vi "TH_Main.vi"() -> ()   [LabVIEW 2014]
uses:
  TH_Ini_Parameters.vi
  TH_Globals.vi
  TH_StartParameters.vi
panel:
  in  "Main Tab Control":T1(tab)
  in  "Visa logbok":bool
  out "Loggbok":string
  out "FuktCluster":T2={"Fukt 1 (%)"=nan, "Fukt 2 (%)"=nan, "Fukt 3 (%)"=nan} {"Fukt 3 (%)" format="%.1f"; "Fukt 2 (%)" format="%.1f"; "Fukt 1 (%)" format="%.1f"}
  out "TempCluster":T3={"Temp 1 (°C)"=nan, "Temp 2 (°C)"=nan, "Temp 3 (°C)"=nan} {"Temp 3 (°C)" format="%.1f"; "Temp 2 (°C)" format="%.1f"; "Temp 1 (°C)" format="%.1f"}
  out "Tid/Datum":string
  out "Read":bool
  out "TimeDateCluster":T4
  out "Tid/Datum Temp":string
  out "Medeltemp 3":dbl=nan format="%.1f"
  out "Medeltemp 2":dbl=nan format="%.1f"
  out "Medeltemp 1":dbl=nan format="%.1f"
  out "TempXY":T5(graph)
  out "Tid/Datum Fukt":string
  out "Medelfukt 3":dbl=nan format="%.1f"
  out "Medelfukt 2":dbl=nan format="%.1f"
  out "Medelfukt 1":dbl=nan format="%.1f"
  out "FuktXY":T5(graph)
  in  "Medelvärdes-\nbildning":u16(ring) items=["Ingen", "Dynamisk", "6 timmar", "24 timmar"]
  in  "Läs in data":bool
  in  "Slut Dag":u16(ring) items=["1", "2", "3", "4", "5", "6", "7", "8", "9", "10", "11", "12", "13", "14", "15", "16", "17", "18", "19", "20", "21", "22", "23", "24", "25", "26", "27", "28", "29", "30", "31"]
  in  "Slut Månad":u16(ring) items=["Januari", "Februari", "Mars", "April", "Maj", "Juni", "Juli", "Augusti", "September", "Oktober", "November", "December"]
  in  "Slut År":u16(ring)=4 items=["2001", "2002", "2003", "2004", "2005", "2006", "2007", "2008", "2009", "2010", "2011", "2012", "2013", "2014", "2015"]
  in  "Start Dag":u16(ring) items=["1", "2", "3", "4", "5", "6", "7", "8", "9", "10", "11", "12", "13", "14", "15", "16", "17", "18", "19", "20", "21", "22", "23", "24", "25", "26", "27", "28", "29", "30", "31"]
  in  "Start Månad":u16(ring) items=["Januari", "Februari", "Mars", "April", "Maj", "Juni", "Juli", "Augusti", "September", "Oktober", "November", "December"]
  in  "Start År":u16(ring)=4 items=["2001", "2002", "2003", "2004", "2005", "2006", "2007", "2008", "2009", "2010", "2011", "2012", "2013", "2014", "2015"]
  out "XY Graph":T6(graph)
  in  "Starta backup":bool
  in  "Backup år":u16(ring)=4 items=["2001", "2002", "2003", "2004", "2005", "2006", "2007", "2008", "2009", "2010"]
  in  "Bladmögel":T7={"Tid (timmar)"=4.0, "Temp (°C)"=3.0, "Fukt (%)"=93.0} {"Fukt (%)" min=0.0 max=100.0 format="%.1f"; "Temp (°C)" min=-25.0 max=85.0 step=0.1 format="%.1f"; "Tid (timmar)" min=0.01 format="%.2f"}
  in  "MainExit":bool
  in  "Skriv ut skärmbild":bool
  # "Från:"
  # "Till:"
  # "Backup av mätdata\ntill diskett A:\\"
  # "Bladmögelvarning\nför givare 1"
  # "TH-Logger är ett svenskutvecklat program som visar och lagrar temperatur och fukt information om förhållandena i vilka lagerutrymmen som helst.\n\nProgrammet är utvecklat av Roine Stenberg och Niklas Jonsson och har varit i drift och utvecklats sedan hösten 2001, bland annat i Niklas Jonssons eget lager på Follinge Krongård.\n\nMer information om programmet och hur det kan användas får du genom att ringa Niklas Jonsson på telefon 0142-41749 eller 0708-441749. Tekniska frågor besvaras av Roine Stenberg på telefon 013-105646 eller 0733-253321.\n\nPå internet finns också en del information om programmet på adressen http://www.follinge.se"
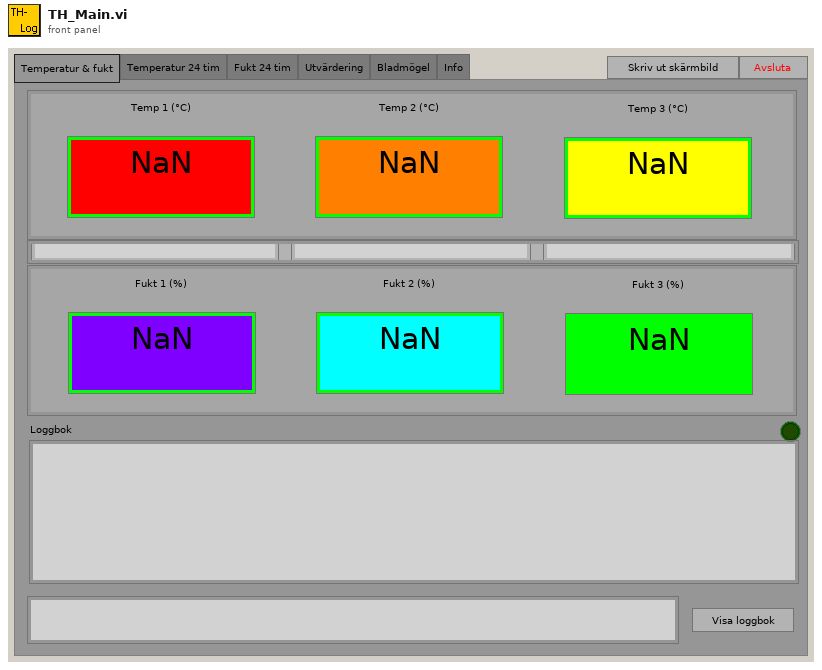
[diagram p1: front panel]
types:
  T1 = enum32{"Temperatur & fukt", "Temperatur 24 tim", "Fukt 24 tim", "Utvärdering", "Bladmögel", "Info"}
  T2 = cluster{"Fukt 1 (%)":dbl, "Fukt 2 (%)":dbl, "Fukt 3 (%)":dbl}
  T3 = cluster{"Temp 1 (°C)":dbl, "Temp 2 (°C)":dbl, "Temp 3 (°C)":dbl}
  T4 = cluster{"TimeDate 1":string, "TimeDate 2":string, "TimeDate 3":string}
  T5 = cluster{"XY chart data":cluster{"x":dbl, "y":dbl}[]}[]
  T6 = cluster{cluster{"Numeric":dbl, "Numeric":dbl}[]}[]
  T7 = cluster{"Tid (timmar)":dbl, "Temp (°C)":dbl, "Fukt (%)":dbl}
  T8 = cluster{"Temperatures[0]":dbl, "Temperatures[1]":dbl, "Temperatures[2]":dbl}
  T9 = cluster{"Humidities[0]":dbl, "Humidities[1]":dbl, "Humidities[2]":dbl}
  T10 = typedef "NH485 Object Reference.ctl" = refnum<k1>
  T11 = cluster{"[0]":string, "[1]":string, "[2]":string}
  T12 = cluster{"Start År":u16, "Start Månad":u16, "Start Dag":u16, "Slut År":u16, "Slut Månad":u16, "Slut Dag":u16}
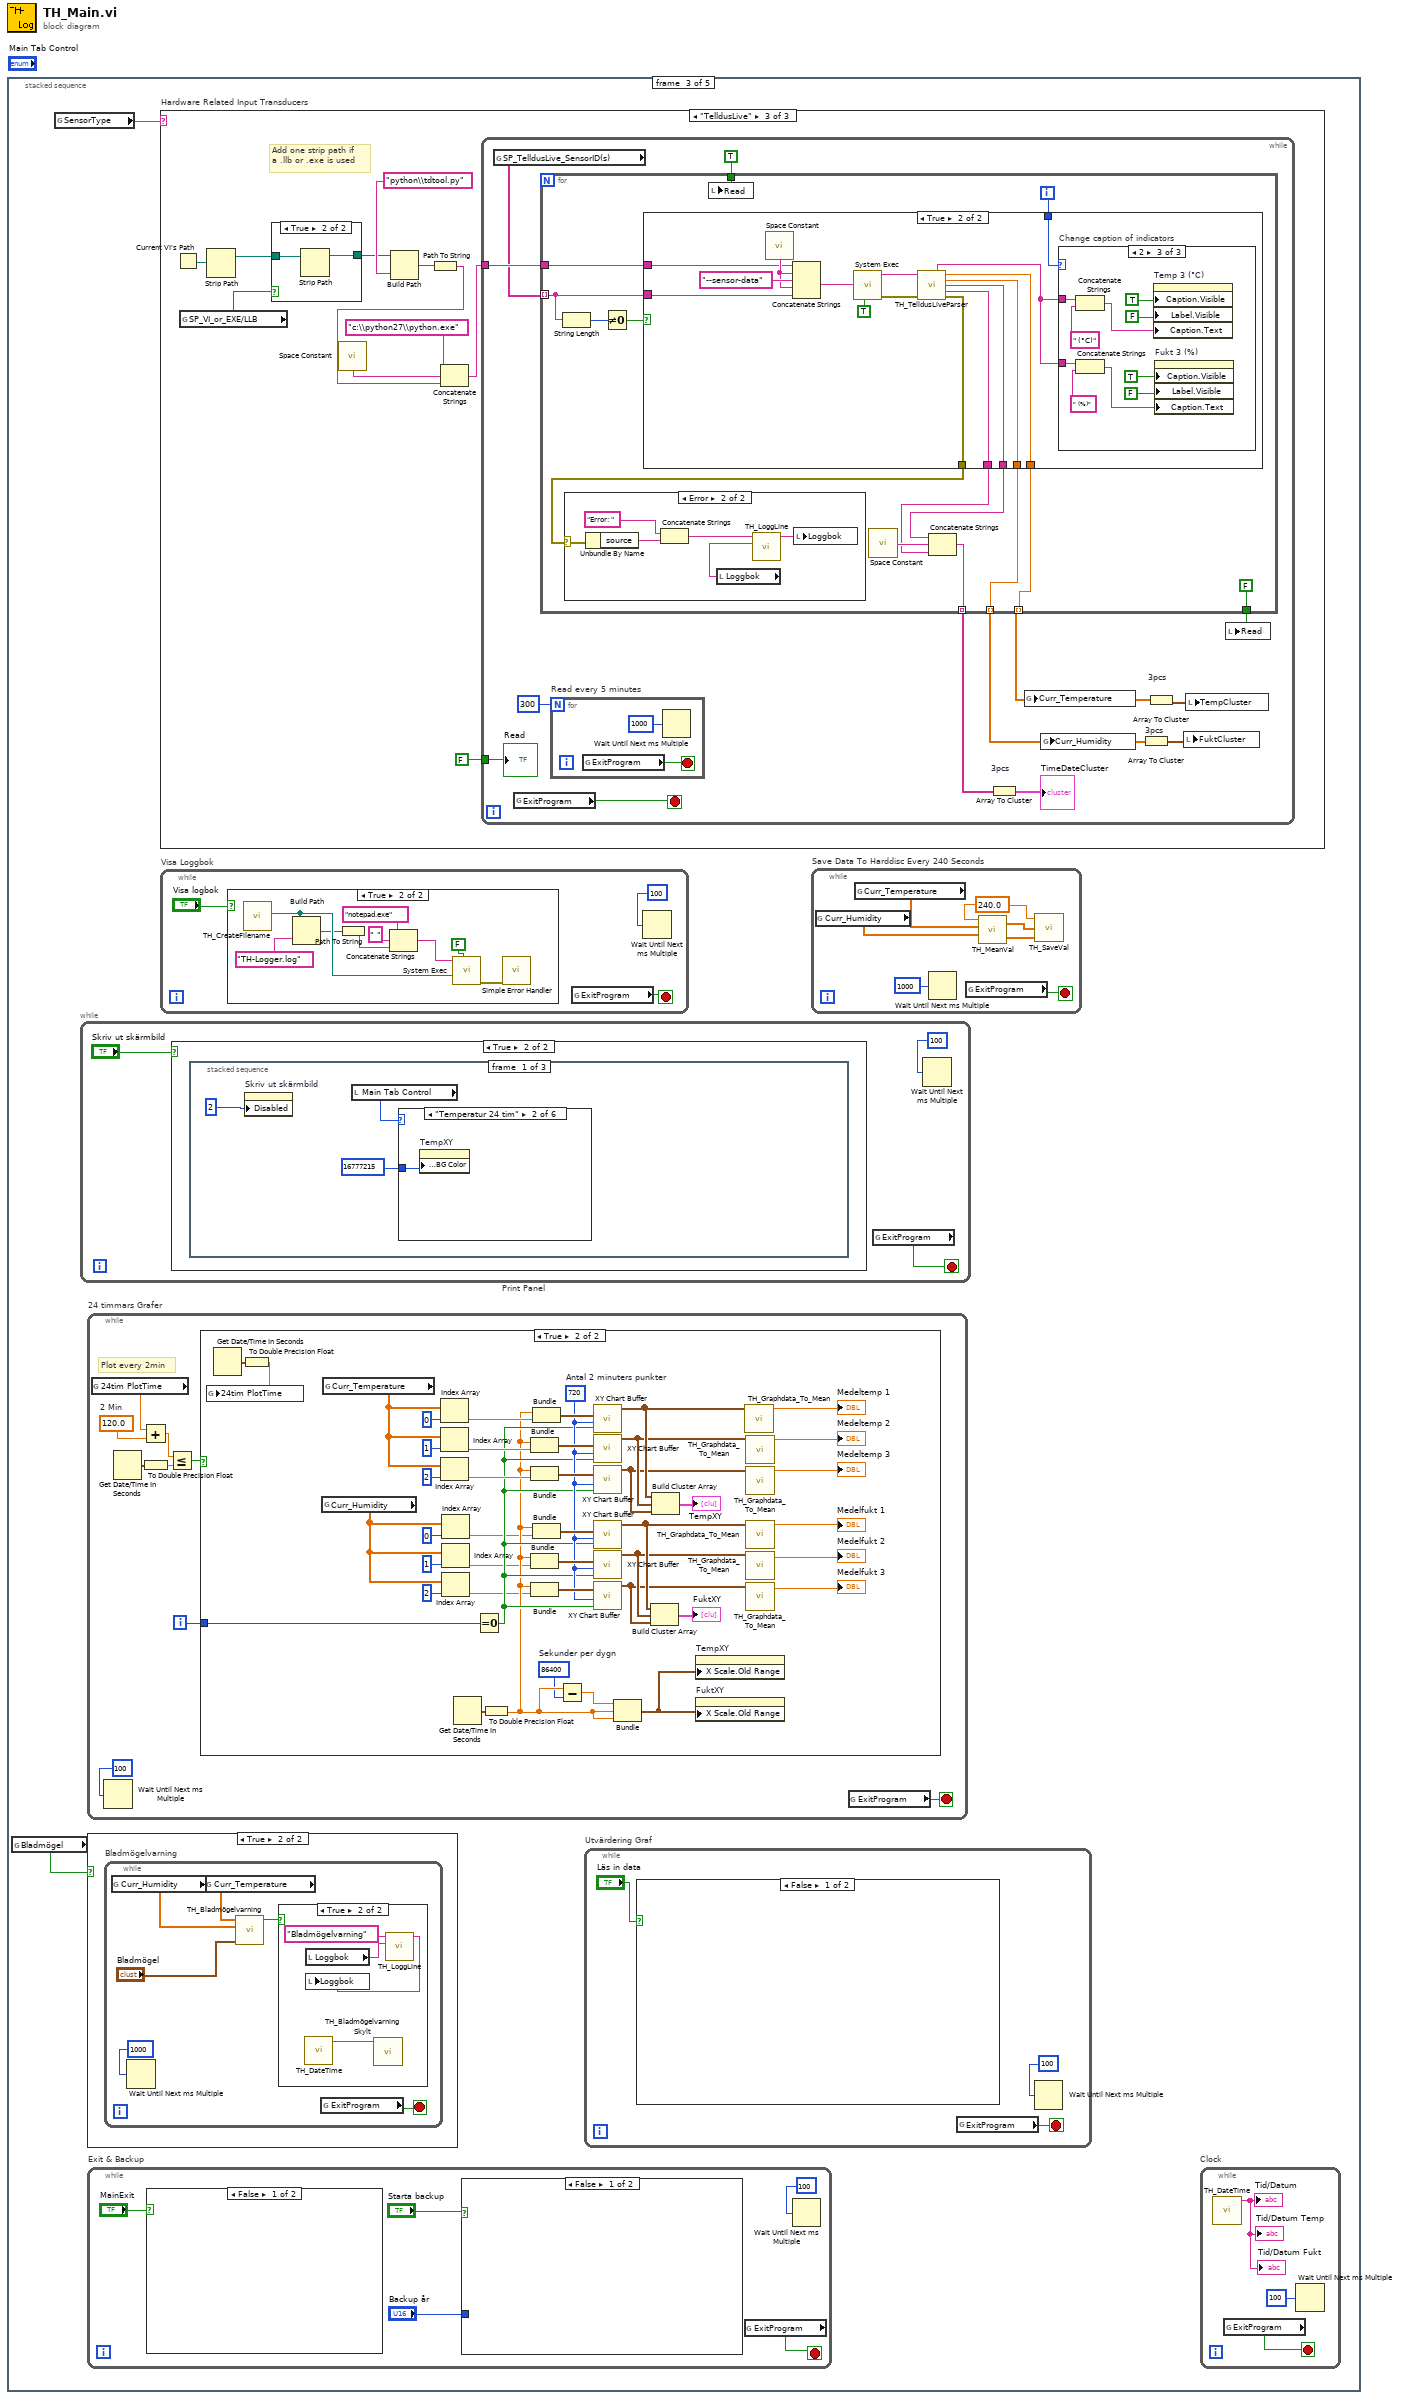
[diagram p0: block diagram]
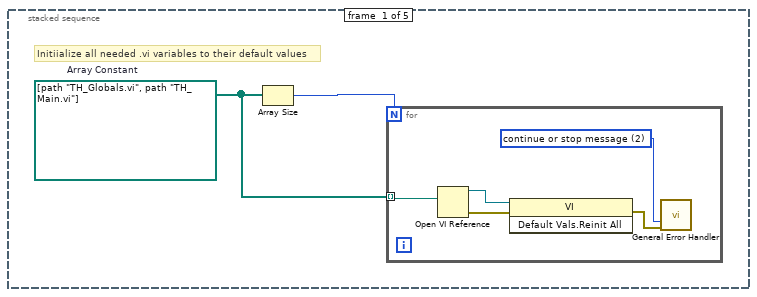
[diagram p2: hidden frame]
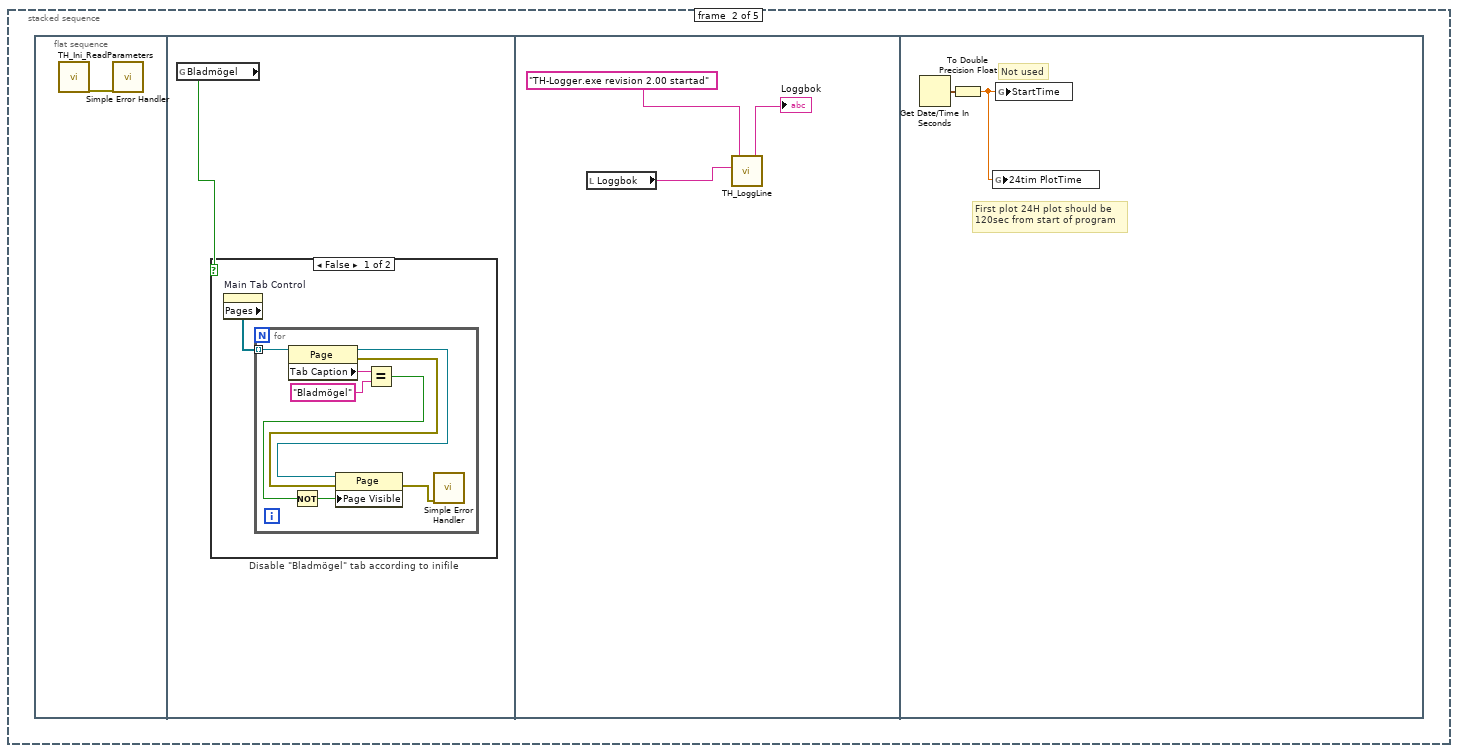
[diagram p3: hidden frame]
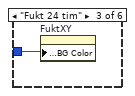
[diagram p10: hidden frame]
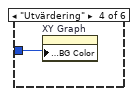
[diagram p11: hidden frame]
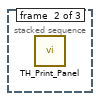
[diagram p14: hidden frame]
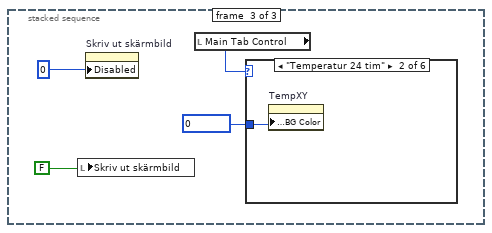
[diagram p15: hidden frame]
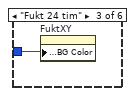
[diagram p17: hidden frame]
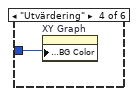
[diagram p18: hidden frame]
diagram:
  n1 = stacked-sequence {
    frame #0 {
      w1 = path[] [path "TH_Globals.vi", path "TH_Main.vi"]  # Array Constant
      # "Initiialize all needed .vi variables to their default values"
      n2 = Array Size(array=w1) -> (size(s)=w2:i32)
      n3 = for {
        N: w2 -> [_]
        tunnel: w1 -> [w7] mode=indexing
        w3 = u16 2 items=["no dialog", "OK message", "continue or stop message"] ("type of dialog (OK msg:1)")
        n4 = Open VI Reference(vi path=w7) -> (vi reference=w5:refnum<vi>, error out=w6:errorcluster)  [unwired: 5 in]
        n5 = invoke class="VI" method="Default Vals.Reinit All"(reference=w5, error in=w6) -> (error out=w4:errorcluster)  [unwired: 1 in, 2 out]
        n6 = call <vilib>:"General Error Handler.vi"("type of dialog (OK msg:1)"=w3, "error in (no error)"=w4) -> ()  [unwired: 9 in, 5 out]
      }
    }
    frame #1 {
      n7 = flat-sequence {
        frame #0 {
          n8 = call "TH_Ini_ReadParameters.vi"() -> ("error out"=w8:errorcluster)  [unwired: 19 in]
          n9 = call <vilib>:"Simple Error Handler.vi"("error in (no error)"=w8) -> ()  [unwired: 4 in, 5 out]
        }
        frame #1 {
          n10 = global read "TH_Ini_Parameters.vi" "Bladmögel"() -> (w9:bool)
          n11 = case "Disable \"Bladmögel\" tab according to inifile" shown="False" w9 {
            frame False {
              n12 = property on="Main Tab Control" class="TabCtl (strict)"() -> ("Pages"=w10:refnum<vi>[])  [unwired: 2 in, 2 out]
              n13 = for {
                tunnel: w10 -> [w18] mode=indexing
                n14 = property class="Page"(reference=w18) -> (reference out=w14:refnum<vi>, error out=w15:errorcluster, "Tab Caption"=w17:string)  [unwired: 1 in]
                n15 = Equal?(x=w17, y="Bladmögel") -> (x = y?=w12:bool)
                n16 = Not(x=w12) -> (.not. x?=w11:bool)
                n17 = property class="Page"(reference=w14, error in=w15, "Page Visible"=w11) -> (error out=w13:errorcluster)  [unwired: 1 out]
                n18 = call <vilib>:"Simple Error Handler.vi"("error in (no error)"=w13) -> ()  [unwired: 4 in, 5 out]
              }
            }
            frame True {
            }
          }
        }
        frame #2 {
          n19 = local read "Loggbok"() -> (w21:string)
          n20 = call "TH_LoggLine.vi"("Händelse Logg In"=w21, "Logg String In"="TH-Logger.exe revision 2.00 startad") -> ("Händelse Logg Out"=→"Loggbok":string)  [unwired: 5 in]
        }
        frame #3 {
          # "Not used"
          # "First plot 24H plot should be\n120sec from start of program"
          n21 = Get Date/Time In Seconds() -> (seconds since 1Jan1904=w23:timestamp)
          n22 = To Double Precision Float(number=w23) -> (double precision float=w22:dbl)
          n23 = global write "TH_Globals.vi" "24tim PlotTime"(w22) -> ()
          n24 = global write "TH_Globals.vi" "StartTime"(w22) -> ()
        }
      }
    }
    frame #2 {
      n25 = global read "TH_Ini_Parameters.vi" "Bladmögel"() -> (w24:bool)
      n26 = global read "TH_Ini_Parameters.vi" "SensorType"() -> (w25:string)
      n27 = while "Print Panel" {
        stop <- w49 stop-if-true
        n28 = case shown="True" "Skriv ut skärmbild" {
          frame False {
          }
          frame True {
            n29 = stacked-sequence {
              frame #0 {
                n30 = property on="Skriv ut skärmbild" class="Bool (strict)"("Disabled"=2) -> ()  [unwired: 2 in, 2 out]
                n31 = local read "Main Tab Control"() -> (w52:T1)
                n32 = case shown="\"Temperatur 24 tim\"" w52 {
                  tunnel: u32 16777215 ("Plot Area:Colors:BG Color") -> [_ w54 w55 w56 _ _]
                  frame "Temperatur & fukt", Default {
                  }
                  frame "Temperatur 24 tim" {
                    n33 = property on="TempXY" class="XYGraph (strict)"("Plot Area:Colors:BG Color"=w54) -> ()  [unwired: 2 in, 2 out]
                  }
                  frame "Fukt 24 tim" {
                    n34 = property on="FuktXY" class="XYGraph (strict)"("Plot Area:Colors:BG Color"=w55) -> ()  [unwired: 2 in, 2 out]
                  }
                  frame "Utvärdering" {
                    n35 = property on="XY Graph" class="XYGraph (strict)"("Plot Area:Colors:BG Color"=w56) -> ()  [unwired: 2 in, 2 out]
                  }
                  frame "Bladmögel" {
                  }
                  frame "Info" {
                  }
                }
              }
              frame #1 {
                n36 = call "TH_Print_Panel.vi"() -> ()  [unwired: 20 in]
              }
              frame #2 {
                n37 = local write "Skriv ut skärmbild"(FALSE) -> ()
                n38 = property on="Skriv ut skärmbild" class="Bool (strict)"("Disabled"=0) -> ()  [unwired: 2 in, 2 out]
                n39 = local read "Main Tab Control"() -> (w58:T1)
                n40 = case shown="\"Temperatur 24 tim\"" w58 {
                  tunnel: u32 0 ("Plot Area:Colors:BG Color") -> [_ w61 w62 w63 _ _]
                  frame "Temperatur & fukt", Default {
                  }
                  frame "Temperatur 24 tim" {
                    n41 = property on="TempXY" class="XYGraph (strict)"("Plot Area:Colors:BG Color"=w61) -> ()  [unwired: 2 in, 2 out]
                  }
                  frame "Fukt 24 tim" {
                    n42 = property on="FuktXY" class="XYGraph (strict)"("Plot Area:Colors:BG Color"=w62) -> ()  [unwired: 2 in, 2 out]
                  }
                  frame "Utvärdering" {
                    n43 = property on="XY Graph" class="XYGraph (strict)"("Plot Area:Colors:BG Color"=w63) -> ()  [unwired: 2 in, 2 out]
                  }
                  frame "Bladmögel" {
                  }
                  frame "Info" {
                  }
                }
              }
            }
          }
        }
        n44 = global read "TH_Globals.vi" "ExitProgram"() -> (w49:bool)
        n45 = Wait Until Next ms Multiple(millisecond multiple=u32 100) -> ()  [unwired: 1 out]
      }
      n46 = while "24 timmars Grafer" {
        i -> [w72]
        stop <- w65 stop-if-true
        w68 = 120.0  # 2 Min
        # "Plot every 2min"
        n47 = global read "TH_Globals.vi" "24tim PlotTime"() -> (w67:dbl)
        n48 = Wait Until Next ms Multiple(millisecond multiple=u32 100) -> ()  [unwired: 1 out]
        n49 = Get Date/Time In Seconds() -> (seconds since 1Jan1904=w64:timestamp)
        n50 = Add(x=w67, y=w68) -> (x+y=w69:dbl)
        n51 = To Double Precision Float(number=w64) -> (double precision float=w70:dbl)
        n52 = Less Or Equal?(x=w69, y=w70) -> (x <= y?=w66:bool)
        n53 = case shown="True" w66 {
          tunnel: w72 -> [_ w116]
          frame False {
          }
          frame True {
            w95 = 720  # Antal 2 minuters punkter
            w88 = 86400  # Sekunder per dygn
            n54 = Get Date/Time In Seconds() -> (seconds since 1Jan1904=w73:timestamp)
            n55 = To Double Precision Float(number=w73) -> (double precision float=w115:dbl)
            n56 = global write "TH_Globals.vi" "24tim PlotTime"(w115) -> ()
            n57 = global read "TH_Globals.vi" "Curr_Humidity"() -> (w99:dbl[])
            n58 = global read "TH_Globals.vi" "Curr_Temperature"() -> (w109:dbl[])
            n59 = Index Array(array=w109, index=0) -> (element=w111:dbl)
            n60 = Index Array(array=w109, index=1) -> (element=w110:dbl)
            n61 = Index Array(array=w109, index=2) -> (element=w105:dbl)
            n62 = Index Array(array=w99, index=0) -> (element=w92:dbl)
            n63 = Index Array(array=w99, index=1) -> (element=w91:dbl)
            n64 = Index Array(array=w99, index=2) -> (element=w90:dbl)
            n65 = Get Date/Time In Seconds() -> (seconds since 1Jan1904=w74:timestamp)
            n66 = Equal To 0?(x=w116) -> (x = 0?=w94:bool)
            n67 = To Double Precision Float(number=w74) -> (double precision float=w93:dbl)
            n68 = Bundle(w93, "Numeric"=w110) -> (w112:cluster{dbl, "Numeric":dbl})  [unwired: 1 in]
            n69 = Bundle(w93, "Numeric"=w105) -> (w103:cluster{dbl, "Numeric":dbl})  [unwired: 1 in]
            n70 = Bundle(w93, "Numeric"=w91) -> (w97:cluster{dbl, "Numeric":dbl})  [unwired: 1 in]
            n71 = Bundle(w93, "Numeric"=w90) -> (w98:cluster{dbl, "Numeric":dbl})  [unwired: 1 in]
            n72 = Bundle(w93, "Numeric"=w111) -> (w114:cluster{dbl, "Numeric":dbl})  [unwired: 1 in]
            n73 = Bundle(w93, "Numeric"=w92) -> (w96:cluster{dbl, "Numeric":dbl})  [unwired: 1 in]
            n74 = Subtract(x=w93, y=w88) -> (x-y=w113:dbl)
            n75 = call "XY Chart Buffer.vi"("clear first (no:F)"=w94, "chart length (points)"=w95, "new point"=w114) -> ("XY chart data"=w86:cluster{"x":dbl, "y":dbl}[])  [unwired: 8 in]
            n76 = call "XY Chart Buffer.vi"("clear first (no:F)"=w94, "chart length (points)"=w95, "new point"=w112) -> ("XY chart data"=w85:cluster{"x":dbl, "y":dbl}[])  [unwired: 8 in]
            n77 = call "XY Chart Buffer.vi"("clear first (no:F)"=w94, "chart length (points)"=w95, "new point"=w103) -> ("XY chart data"=w84:cluster{"x":dbl, "y":dbl}[])  [unwired: 8 in]
            n78 = call "XY Chart Buffer.vi"("clear first (no:F)"=w94, "chart length (points)"=w95, "new point"=w96) -> ("XY chart data"=w83:cluster{"x":dbl, "y":dbl}[])  [unwired: 8 in]
            n79 = call "XY Chart Buffer.vi"("clear first (no:F)"=w94, "chart length (points)"=w95, "new point"=w97) -> ("XY chart data"=w82:cluster{"x":dbl, "y":dbl}[])  [unwired: 8 in]
            n80 = call "XY Chart Buffer.vi"("clear first (no:F)"=w94, "chart length (points)"=w95, "new point"=w98) -> ("XY chart data"=w81:cluster{"x":dbl, "y":dbl}[])  [unwired: 8 in]
            n81 = Bundle(w113, w93, w93) -> (w87:cluster{dbl, dbl, dbl})  [unwired: 1 in]
            n82 = Build Cluster Array(w83, w82, w81) -> (→"FuktXY":T5)
            n83 = Build Cluster Array(w86, w85, w84) -> (→"TempXY":T5)
            n84 = property on="TempXY" class="XYGraph (strict)"("X Scale.Old Range"=w87) -> ()  [unwired: 2 in, 2 out]
            n85 = property on="FuktXY" class="XYGraph (strict)"("X Scale.Old Range"=w87) -> ()  [unwired: 2 in, 2 out]
            n86 = call "TH_Graphdata_To_Mean.vi"("XY chart data"=w86) -> ("MeanValue"=→"Medeltemp 1":dbl)  [unwired: 5 in, 1 out]
            n87 = call "TH_Graphdata_To_Mean.vi"("XY chart data"=w85) -> ("MeanValue"=→"Medeltemp 2":dbl)  [unwired: 5 in, 1 out]
            n88 = call "TH_Graphdata_To_Mean.vi"("XY chart data"=w84) -> ("MeanValue"=→"Medeltemp 3":dbl)  [unwired: 5 in, 1 out]
            n89 = call "TH_Graphdata_To_Mean.vi"("XY chart data"=w83) -> ("MeanValue"=→"Medelfukt 1":dbl)  [unwired: 5 in, 1 out]
            n90 = call "TH_Graphdata_To_Mean.vi"("XY chart data"=w82) -> ("MeanValue"=→"Medelfukt 2":dbl)  [unwired: 5 in, 1 out]
            n91 = call "TH_Graphdata_To_Mean.vi"("XY chart data"=w81) -> ("MeanValue"=→"Medelfukt 3":dbl)  [unwired: 5 in, 1 out]
          }
        }
        n92 = global read "TH_Globals.vi" "ExitProgram"() -> (w65:bool)
      }
      n93 = case shown="True" w24 {
        frame False {
        }
        frame True {
          n94 = while "Bladmögelvarning" {
            stop <- w27 stop-if-true
            n95 = global read "TH_Globals.vi" "Curr_Humidity"() -> (w29:dbl[])
            n96 = Wait Until Next ms Multiple(millisecond multiple=u32 1000) -> ()  [unwired: 1 out]
            n97 = global read "TH_Globals.vi" "Curr_Temperature"() -> (w30:dbl[])
            n98 = call "TH_Bladmögelvarning.vi"("Bladmögelvarning"="Bladmögel", "Humidities In"=w29, "Temperatures In"=w30) -> ("Bladmägelvarning (T/F)"=w26:bool)  [unwired: 4 in]
            n99 = case shown="True" w26 {
              frame False {
              }
              frame True {
                n100 = call "TH_DateTime.vi"() -> ("Tid och Datum"=w32:string)  [unwired: 7 in]
                n101 = local read "Loggbok"() -> (w33:string)
                n102 = call "TH_Bladmögelvarning Skylt.vi"("Tid"=w32) -> ()  [unwired: 7 in]
                n103 = call "TH_LoggLine.vi"("Händelse Logg In"=w33, "Logg String In"="Bladmögelvarning") -> ("Händelse Logg Out"=w35:string)  [unwired: 5 in]
                n104 = local write "Loggbok"(w35) -> ()
              }
            }
            n105 = global read "TH_Globals.vi" "ExitProgram"() -> (w27:bool)
          }
        }
      }
      n106 = while "Exit & Backup" {
        stop <- w136 stop-if-true
        n107 = case shown="False" "MainExit" {
          frame False {
          }
          frame True {
            n108 = Two Button Dialog(message="Är du säker på att du vill avsluta detta program?", 1:"Nej" ("F button name (\"Cancel\")"), 2:"Ja" ("T button name (\"OK\")")) -> (T button?=w152:bool)
            n109 = case shown="True" w152 {
              frame False {
              }
              frame True {
                n110 = global write "TH_Globals.vi" "ExitProgram"(TRUE) -> ()
              }
            }
          }
        }
        n111 = case shown="False" "Starta backup" {
          tunnel: "Backup år" -> [_ w139]
          frame False {
          }
          frame True {
            (unwired) "\u001b" ("message")
            n112 = stacked-sequence {
              tunnel: w139 -> [_ w141 _]
              frame #0 {
                n113 = property on="Starta backup" class="Bool (strict)"("Disabled"=2) -> ()  [unwired: 2 in, 2 out]
              }
              frame #1 {
                n114 = Two Button Dialog(message="Placera en formaterad 1.44MB diskett i diskettstation A:\\\nAlla befintliga filer kommer att raderas!", 1:"Avbryt" ("F button name (\"Cancel\")"), 2:"OK" ("T button name (\"OK\")")) -> (T button?=w142:bool)
                n115 = case shown="True" w142 {
                  tunnel: w141 -> [_ w146]
                  frame False {
                  }
                  frame True {
                    n116 = call "TH_DataBackup.vi"("Backup År"=w146) -> ()  [unwired: 5 in, 2 out]
                  }
                }
              }
              frame #2 {
                n117 = local write "Starta backup"(FALSE) -> ()
                n118 = property on="Starta backup" class="Bool (strict)"("Disabled"=0) -> ()  [unwired: 2 in, 2 out]
              }
            }
          }
        }
        n119 = global read "TH_Globals.vi" "ExitProgram"() -> (w136:bool)
        n120 = Wait Until Next ms Multiple(millisecond multiple=u32 100) -> ()  [unwired: 1 out]
      }
      n121 = case "Hardware Related Input Transducers" shown="\"TelldusLive\"" w25 {
        frame "HygroWin", Default {
          n122 = global read "TH_StartParameters.vi" "SP_HygroWin_COMport(s)"() -> (w165:refnum<visa-resource-name>[])
          n123 = call "TH_RS232_Init.vi"("COMports"=w165) -> ("error out array"=w164:errorcluster[], "COMhandles"=w168:refnum<visa-resource-name>[])  [unwired: 5 in]
          n124 = while "Read Port Loop (This should be the fastest routine in the program)" {
            tunnel: [w170] -> w166
            tunnel: w164 -> [w174]
            tunnel: [w177] -> w167
            tunnel: w168 -> [w178]
            stop <- w169 stop-if-true
            n125 = call "TH_RS232_Read.vi"("COMhandles In"=w178, "error in array"=w174) -> ("NewValues Out"=w173:bool[], "COMhandles Out"=w177:refnum<visa-resource-name>[], "Temperatures"=w171:dbl[], "Humidities"=w172:dbl[], "error out array"=w170:errorcluster[])  [unwired: 2 in]
            n126 = global write "TH_Globals.vi" "Curr_Temperature"(w171) -> ()
            n127 = Array To Cluster "3pcs"(array=w171) -> (cluster=→"TempCluster":T8)
            n128 = global write "TH_Globals.vi" "Curr_Humidity"(w172) -> ()
            n129 = global write "TH_Globals.vi" "NewValues"(w173) -> ()
            n130 = Array To Cluster "3pcs"(array=w172) -> (cluster=→"FuktCluster":T9)
            n131 = global read "TH_Globals.vi" "ExitProgram"() -> (w169:bool)
            n132 = Wait Until Next ms Multiple(millisecond multiple=u32 100) -> ()  [unwired: 1 out]
          }
          n133 = for "Create/Open Error Dialog" {
            tunnel: w164 -> [w181] mode=indexing
            i -> [w180]
            n134 = case shown="Error" w181 {
              tunnel: w180 -> [_ w186]
              frame No Error {
              }
              frame Error {
                n135 = Number To Decimal String(number=w186) -> (decimal integer string=w185:string)  [unwired: 1 in]
                n136 = local read "Loggbok"() -> (w184:string)
                n137 = Concatenate Strings("Error, Open VISA Port. Array Position ", w185) -> (w182:string)
                n138 = call "TH_LoggLine.vi"("Händelse Logg In"=w184, "Logg String In"=w182) -> ("Händelse Logg Out"=w183:string)  [unwired: 5 in]
                n139 = local write "Loggbok"(w183) -> ()
              }
            }
          }
          n140 = call "TH_RS232_Exit.vi"("Array"=w166, "COMports"=w167) -> ()  [unwired: 6 in]
        }
        frame "NH485" {
          n141 = global read "TH_StartParameters.vi" "SP_NH485_COMport"() -> (w189:refnum<visa-resource-name>[])
          n142 = global read "TH_StartParameters.vi" "SP_NH485_Adress(es)"() -> (w188:u32[])
          n143 = for "Create/Open" {
            tunnel: w189 -> [w234] mode=indexing
            tunnel: [w231] -> w190 mode=indexing
            tunnel: [w230] -> w191 mode=indexing
            tunnel: w188 -> [w229] mode=indexing
            n144 = call "NH485 Create.vi"("Address"=w229, "VISA Resource Name"=w234) -> ("error out"=w232:errorcluster, "reference"=w233:T10)  [unwired: 4 in]
            n145 = call "NH485 Open.vi"("error in (no error)"=w232, "reference"=w233) -> ("error out"=w230:errorcluster, "duplicate reference"=w231:T10)  [unwired: 8 in]
          }
          n146 = for "Create/Open Error Dialog" {
            tunnel: w191 -> [w218] mode=indexing
            i -> [w217]
            n147 = case shown="Error" w218 {
              tunnel: w217 -> [_ w223]
              frame No Error {
              }
              frame Error {
                n148 = Number To Decimal String(number=w223) -> (decimal integer string=w222:string)  [unwired: 1 in]
                n149 = local read "Loggbok"() -> (w221:string)
                n150 = Concatenate Strings("Error, Open VISA Port. Array Position ", w222) -> (w219:string)
                n151 = call "TH_LoggLine.vi"("Händelse Logg In"=w221, "Logg String In"=w219) -> ("Händelse Logg Out"=w220:string)  [unwired: 5 in]
                n152 = local write "Loggbok"(w220) -> ()
              }
            }
          }
          n153 = while "Read Transducer Data" {
            tunnel: [w195] -> w192
            tunnel: [w196] -> w193
            tunnel: w191 -> [w198]
            tunnel: w190 -> [w199]
            stop <- w194 stop-if-true
            n154 = for {
              tunnel: [w204] -> w195 mode=indexing
              tunnel: [w203] -> w196 mode=indexing
              tunnel: w199 -> [w202] mode=indexing
              tunnel: w198 -> [w201] mode=indexing
              n155 = call "NH485 Measure.vi"("error in (no error)"=w201, "reference"=w202) -> ("error out"=w204:errorcluster, "duplicate reference"=w203:T10)  [unwired: 8 in]
              n156 = Wait (ms)(milliseconds to wait=200) -> ()  [unwired: 1 out]
            }
            n157 = global read "TH_Globals.vi" "ExitProgram"() -> (w194:bool)
            n158 = Wait Until Next ms Multiple(millisecond multiple=u32 2000) -> ()  [unwired: 1 out]
          }
          n159 = while "GUI & Global Variable Store" {
            tunnel: w190 -> [w210]
            tunnel: w191 -> [w211]
            stop <- w209 stop-if-true
            n160 = for {
              tunnel: w211 -> [w216] mode=indexing
              tunnel: w210 -> [w215] mode=indexing
              tunnel: [w214] -> w206 mode=indexing
              tunnel: [w213] -> w205 mode=indexing
              n161 = call "NH485 Read.vi"("error in (no error)"=w216, "reference"=w215) -> ("Humidity"=w213:dbl, "Temp"=w214:dbl)  [unwired: 6 in, 2 out]
            }
            n162 = global write "TH_Globals.vi" "Curr_Temperature"(w206) -> ()
            n163 = Array To Cluster "3pcs"(array=w206) -> (cluster=w208:cluster{"[0]":dbl, "[1]":dbl, "[2]":dbl})
            n164 = local write "TempCluster"(w208) -> ()
            n165 = global read "TH_Globals.vi" "ExitProgram"() -> (w209:bool)
            n166 = global write "TH_Globals.vi" "Curr_Humidity"(w205) -> ()
            n167 = Array To Cluster "3pcs"(array=w205) -> (cluster=w207:cluster{"[0]":dbl, "[1]":dbl, "[2]":dbl})
            n168 = local write "FuktCluster"(w207) -> ()
            n169 = Wait Until Next ms Multiple(millisecond multiple=u32 1000) -> ()  [unwired: 1 out]
          }
          n170 = for "Close/Destory" {
            tunnel: w193 -> [w228] mode=indexing
            tunnel: w192 -> [w227] mode=indexing
            n171 = call "NH485 Close.vi"("error in (no error)"=w227, "reference"=w228) -> ("error out"=w226:errorcluster, "duplicate reference"=w225:T10)  [unwired: 8 in]
            n172 = call "NH485 Destroy.vi"("error in (no error)"=w226, "reference"=w225) -> ()  [unwired: 5 in, 1 out]
          }
        }
        frame "TelldusLive" {
          # "Add one strip path if\na .llb or .exe is used"
          n173 = Current VI's Path() -> (path=w242:path)
          n174 = global read "TH_StartParameters.vi" "SP_VI_or_EXE/LLB"() -> (w244:bool)
          n175 = Strip Path(path=w242) -> (stripped path=w241:path)  [unwired: 1 out]
          n176 = case shown="True" w244 {
            tunnel: w241 -> [w246 w248]
            tunnel: [w246 w247] -> w243
            frame False {
            }
            frame True {
              n177 = Strip Path(path=w248) -> (stripped path=w247:path)  [unwired: 1 out]
            }
          }
          n178 = call <vilib>:"Space Constant.vi"() -> ("String"=w238:string)
          n179 = Build Path(base path=w243, name or relative path="python\\tdtool.py") -> (appended path=w240:path)
          n180 = Path To String(path=w240) -> (string=w237:string)
          n181 = Concatenate Strings("c:\\python27\\python.exe", w238, w237) -> (w236:string)
          n182 = while {
            tunnel: w236 -> [w261]
            tunnel: FALSE ("Read") -> [w257]
            stop <- w254 stop-if-true
            n183 = global read "TH_StartParameters.vi" "SP_TelldusLive_SensorID(s)"() -> (w260:string[])
            n184 = global read "TH_Globals.vi" "ExitProgram"() -> (w254:bool)
            n185 = for {
              tunnel: w261 -> [w277]
              tunnel: w260 -> [w270] mode=indexing
              tunnel: [w275] -> w252 mode=indexing
              tunnel: [w276] -> w258 mode=indexing
              tunnel: TRUE ("Read") -> [w272]
              tunnel: [FALSE ("Read")] -> w255
              tunnel: [w264] -> w249 mode=indexing
              i -> [w268]
              n186 = String Length(string=w270) -> (length=w274:i32)
              n187 = Not Equal To 0?(x=w274) -> (x != 0?=w273:bool)
              n188 = case shown="True" w273 {
                tunnel: w277 -> [_ w315]
                tunnel: [errorcluster {"status"=FALSE, "code"=0, "source"=""} ("error constant") w312] -> w269
                tunnel: [w288 w309] -> w276
                tunnel: [w288 w308] -> w275
                tunnel: w270 -> [_ w310]
                tunnel: [w286 w307] -> w267
                tunnel: [w286 w306] -> w265
                tunnel: w268 -> [w285 w305]
                frame False {
                  w286 = ""
                  w288 = nan
                  n189 = case "Change caption of indicators" shown="0, Default" w285 {
                    tunnel: "Not Connected" -> [w289 w294 w299]
                    frame 0, Default {
                      n190 = property on="Fukt 1 (%)" class="DigNum (strict)"("Caption.Visible"=TRUE, "Label.Visible"=FALSE, "Caption.Text"=w289) -> ()  [unwired: 2 in, 2 out]
                      n191 = property on="Temp 1 (°C)" class="DigNum (strict)"("Caption.Visible"=TRUE, "Label.Visible"=FALSE, "Caption.Text"=w289) -> ()  [unwired: 2 in, 2 out]
                    }
                    frame 1 {
                      n192 = property on="Temp 2 (°C)" class="DigNum (strict)"("Caption.Visible"=TRUE, "Label.Visible"=FALSE, "Caption.Text"=w294) -> ()  [unwired: 2 in, 2 out]
                      n193 = property on="Fukt 2 (%)" class="DigNum (strict)"("Caption.Visible"=TRUE, "Label.Visible"=FALSE, "Caption.Text"=w294) -> ()  [unwired: 2 in, 2 out]
                    }
                    frame 2 {
                      n194 = property on="Temp 3 (°C)" class="DigNum (strict)"("Caption.Visible"=TRUE, "Label.Visible"=FALSE, "Caption.Text"=w299) -> ()  [unwired: 2 in, 2 out]
                      n195 = property on="Fukt 3 (%)" class="DigNum (strict)"("Caption.Visible"=TRUE, "Label.Visible"=FALSE, "Caption.Text"=w299) -> ()  [unwired: 2 in, 2 out]
                    }
                  }
                }
                frame True {
                  n196 = call <vilib>:"Space Constant.vi"() -> ("String"=w317:string)
                  n197 = Concatenate Strings(w315, w317, "--sensor-data" ("string"), w317, w310) -> (w316:string)
                  n198 = call <vilib>:"System Exec.vi"("run minimized? (F)"=TRUE, "command line"=w316) -> ("error out"=w311:errorcluster, "standard output"=w313:string)  [unwired: 6 in, 2 out]
                  n199 = call "TH_TelldusLiveParser.vi"("Telldus Sensor String"=w313, "error in (no error)"=w311) -> ("Name"=w304:string, "Temperature"=w308:dbl, "Humidity"=w309:dbl, "Date"=w307:string, "Time"=w306:string, "error out"=w312:errorcluster)  [unwired: 8 in]
                  n200 = case "Change caption of indicators" shown="2" w305 {
                    tunnel: w304 -> [w327 w337 w347]
                    tunnel: w304 -> [w323 w336 w346]
                    frame 0, Default {
                      n201 = Concatenate Strings(w327, " (°C)") -> (w326:string)
                      n202 = Concatenate Strings(w323, " (%)") -> (w322:string)
                      n203 = property on="Fukt 1 (%)" class="DigNum (strict)"("Caption.Visible"=TRUE, "Label.Visible"=FALSE, "Caption.Text"=w322) -> ()  [unwired: 2 in, 2 out]
                      n204 = property on="Temp 1 (°C)" class="DigNum (strict)"("Caption.Visible"=TRUE, "Label.Visible"=FALSE, "Caption.Text"=w326) -> ()  [unwired: 2 in, 2 out]
                    }
                    frame 1 {
                      n205 = Concatenate Strings(w337, " (°C)") -> (w334:string)
                      n206 = Concatenate Strings(w336, " (%)") -> (w331:string)
                      n207 = property on="Temp 2 (°C)" class="DigNum (strict)"("Caption.Visible"=TRUE, "Label.Visible"=FALSE, "Caption.Text"=w334) -> ()  [unwired: 2 in, 2 out]
                      n208 = property on="Fukt 2 (%)" class="DigNum (strict)"("Caption.Visible"=TRUE, "Label.Visible"=FALSE, "Caption.Text"=w331) -> ()  [unwired: 2 in, 2 out]
                    }
                    frame 2 {
                      n209 = Concatenate Strings(w347, " (°C)") -> (w342:string)
                      n210 = Concatenate Strings(w346, " (%)") -> (w341:string)
                      n211 = property on="Temp 3 (°C)" class="DigNum (strict)"("Caption.Visible"=TRUE, "Label.Visible"=FALSE, "Caption.Text"=w342) -> ()  [unwired: 2 in, 2 out]
                      n212 = property on="Fukt 3 (%)" class="DigNum (strict)"("Caption.Visible"=TRUE, "Label.Visible"=FALSE, "Caption.Text"=w341) -> ()  [unwired: 2 in, 2 out]
                    }
                  }
                }
              }
              n213 = case shown="Error" w269 {
                selector: w269 -> [_ w281]
                frame No Error {
                }
                frame Error {
                  n214 = Unbundle By Name(w281) -> ("source"=w280:string)
                  n215 = Concatenate Strings("Error: ", w280) -> (w278:string)
                  n216 = local read "Loggbok"() -> (w282:string)
                  n217 = call "TH_LoggLine.vi"("Händelse Logg In"=w282, "Logg String In"=w278) -> ("Händelse Logg Out"=w283:string)  [unwired: 5 in]
                  n218 = local write "Loggbok"(w283) -> ()
                }
              }
              n219 = local write "Read"(w272) -> ()
              n220 = call <vilib>:"Space Constant.vi"() -> ("String"=w266:string)
              n221 = Concatenate Strings(w267, w266, w265) -> (w264:string)
            }
            n222 = for "Read every 5 minutes" {
              N: 300 -> [_]
              stop <- w263 stop-if-true
              n223 = global read "TH_Globals.vi" "ExitProgram"() -> (w263:bool)
              n224 = Wait Until Next ms Multiple(millisecond multiple=u32 1000) -> ()  [unwired: 1 out]
            }
            n225 = Array To Cluster "3pcs"(array=w249) -> (cluster=→"TimeDateCluster":T11)
            n226 = global write "TH_Globals.vi" "Curr_Temperature"(w252) -> ()
            n227 = global write "TH_Globals.vi" "Curr_Humidity"(w258) -> ()
            n228 = Array To Cluster "3pcs"(array=w258) -> (cluster=w259:cluster{"[0]":dbl, "[1]":dbl, "[2]":dbl})
            n229 = Array To Cluster "3pcs"(array=w252) -> (cluster=w251:cluster{"[0]":dbl, "[1]":dbl, "[2]":dbl})
            n230 = local write "FuktCluster"(w259) -> ()
            n231 = local write "TempCluster"(w251) -> ()
            n232 = local write "Read"(w255) -> ()
            "Read" <- w257
          }
        }
      }
      n233 = while "Visa Loggbok" {
        stop <- w37 stop-if-true
        n234 = case shown="True" "Visa logbok" {
          frame False {
          }
          frame True {
            n235 = call "TH_CreateFilename.vi"() -> ("RootPath"=w45:path)  [unwired: 5 in, 2 out]
            n236 = Build Path(base path=w45, name or relative path="TH-Logger.log") -> (appended path=w44:path)
            n237 = Path To String(path=w44) -> (string=w42:string)
            n238 = Concatenate Strings("notepad.exe" ("command line"), " ", w42) -> (w40:string)
            n239 = call <vilib>:"System Exec.vi"("wait until completion? (T)"=FALSE, "working directory"=w45, "command line"=w40) -> ("error out"=w39:errorcluster)  [unwired: 5 in, 3 out]
            n240 = call <vilib>:"Simple Error Handler.vi"("error in (no error)"=w39) -> ()  [unwired: 4 in, 5 out]
          }
        }
        n241 = global read "TH_Globals.vi" "ExitProgram"() -> (w37:bool)
        n242 = Wait Until Next ms Multiple(millisecond multiple=u32 100) -> ()  [unwired: 1 out]
      }
      n243 = while "Utvärdering Graf" {
        stop <- w117 stop-if-true
        n244 = case shown="False" "Läs in data" {
          frame False {
          }
          frame True {
            n245 = stacked-sequence {
              frame #0 {
                n246 = property on="Läs in data" class="Bool (strict)"("Disabled"=2) -> ()  [unwired: 2 in, 2 out]
              }
              frame #1 {
                n247 = Bundle("Start År"="Start År", "Start Månad"="Start Månad", "Start Dag"="Start Dag", "Slut År"="Slut År", "Slut Månad"="Slut Månad", "Slut Dag"="Slut Dag") -> (w125:T12)  [unwired: 1 in]
                n248 = call "TH_Utvärdering.vi"("Medelvärdes-\nbildning"="Medelvärdes-\nbildning", "Input Dates"=w125) -> ("Min-X"=w123:dbl, "Max-X"=w124:dbl, "XY Graph"=→"XY Graph":T6)  [unwired: 3 in]
                n249 = property on="XY Graph" class="XYGraph (strict)"("X Scale.Range:Maximum"=w124) -> ()  [unwired: 2 in, 2 out]
                n250 = property on="XY Graph" class="XYGraph (strict)"("X Scale.Range:Minimum"=w123) -> ()  [unwired: 2 in, 2 out]
              }
              frame #2 {
                n251 = local write "Läs in data"(FALSE) -> ()
                n252 = property on="Läs in data" class="Bool (strict)"("Disabled"=0) -> ()  [unwired: 2 in, 2 out]
              }
            }
          }
        }
        n253 = global read "TH_Globals.vi" "ExitProgram"() -> (w117:bool)
        n254 = Wait Until Next ms Multiple(millisecond multiple=u32 100) -> ()  [unwired: 1 out]
      }
      n255 = while "Save Data To Harddisc Every 240 Seconds" {
        stop <- w160 stop-if-true
        w163 = 240.0 ("MeanTime (sec)")
        n256 = global read "TH_Globals.vi" "Curr_Humidity"() -> (w158:dbl[])
        n257 = global read "TH_Globals.vi" "Curr_Temperature"() -> (w159:dbl[])
        n258 = Wait Until Next ms Multiple(millisecond multiple=u32 1000) -> ()  [unwired: 1 out]
        n259 = global read "TH_Globals.vi" "ExitProgram"() -> (w160:bool)
        n260 = call "TH_MeanVal.vi"("Humidities In"=w158, "Temperatures In"=w159, "MeanTime (sec)"=w163) -> ("MeanHum"=w162:dbl[], "MeanTemp"=w161:dbl[])  [unwired: 1 in]
        n261 = call "TH_SaveVal.vi"("Humidities In"=w162, "Temperatures In"=w161, "MeanTime (sec)"=w163) -> ()
      }
      n262 = while "Clock" {
        stop <- w156 stop-if-true
        n263 = call "TH_DateTime.vi"() -> ("Tid och Datum"=→"Tid/Datum" →"Tid/Datum Temp" →"Tid/Datum Fukt":string)  [unwired: 7 in]
        n264 = global read "TH_Globals.vi" "ExitProgram"() -> (w156:bool)
        n265 = Wait Until Next ms Multiple(millisecond multiple=u32 100) -> ()  [unwired: 1 out]
      }
    }
    frame #3 {
      n266 = flat-sequence {
        frame #0 {
          w349 = TRUE
          w350 = FALSE
          n267 = global read "TH_Ini_Parameters.vi" "Bladmögel"() -> (w351:bool)
          n268 = property on="Temp 1 (°C)" class="DigNum (strict)"("Caption.Visible"=w350, "Label.Visible"=w349) -> ()  [unwired: 2 in, 2 out]
          n269 = property on="Fukt 1 (%)" class="DigNum (strict)"("Caption.Visible"=w350, "Label.Visible"=w349) -> ()  [unwired: 2 in, 2 out]
          n270 = property on="Temp 2 (°C)" class="DigNum (strict)"("Caption.Visible"=w350, "Label.Visible"=w349) -> ()  [unwired: 2 in, 2 out]
          n271 = property on="Fukt 2 (%)" class="DigNum (strict)"("Caption.Visible"=w350, "Label.Visible"=w349) -> ()  [unwired: 2 in, 2 out]
          n272 = property on="Temp 3 (°C)" class="DigNum (strict)"("Caption.Visible"=w350, "Label.Visible"=w349) -> ()  [unwired: 2 in, 2 out]
          n273 = property on="Fukt 3 (%)" class="DigNum (strict)"("Caption.Visible"=w350, "Label.Visible"=w349) -> ()  [unwired: 2 in, 2 out]
          n274 = case "Disable \"Bladmögel\" tab according to inifile" shown="False" w351 {
            frame False {
              n275 = property on="Main Tab Control" class="TabCtl (strict)"() -> ("Pages"=w352:refnum<vi>[])  [unwired: 2 in, 2 out]
              n276 = for {
                tunnel: w352 -> [w355] mode=indexing
                n277 = property class="Page"(reference=w355, "Page Visible"=TRUE) -> (error out=w353:errorcluster)  [unwired: 1 in, 1 out]
                n278 = call <vilib>:"Simple Error Handler.vi"("error in (no error)"=w353) -> ()  [unwired: 4 in, 5 out]
              }
            }
            frame True {
            }
          }
        }
        frame #1 {
          n279 = local read "Loggbok"() -> (w357:string)
          n280 = call "TH_LoggLine.vi"("Händelse Logg In"=w357, "Logg String In"="TH-Logger.exe avslutad") -> ("Händelse Logg Out"=w358:string)  [unwired: 5 in]
          n281 = local write "Loggbok"(w358) -> ()
        }
      }
    }
    frame #4 {
      n282 = global read "TH_StartParameters.vi" "SP_VI_or_EXE/LLB"() -> (w359:bool)
      n283 = Quit LabVIEW(quit? (T)=w359) -> ()
    }
  }
